vi "haotian_sheet_resistance.vi"() -> ()   [LabVIEW 2024]
uses:
  <vilib>/Utility/file.llb/Write Delimited Spreadsheet (DBL).vi
panel:
  out "Device 1 resistance":dbl=36696923.98728005
  out "Ch 1 phase":dbl=6.260435993401659 caption="Device1 phase" format="%.3p"
  out "Device1 Current(uA)":dbl=2.609667211877282
  in  "R1(Kohm)":dbl=2000.0 format="%#_13g"
  in  "path2 (folder + filename)":string="H:\\My Drive\\Lab\\PPMS\\Measurement\\GaN_1000C_3min_1314_1112"
  in  "Save data or not":bool=TRUE
  in  "path1 (folder + filename)":string="H:\\My Drive\\Lab\\PPMS\\Measurement\\GaN_1000C_2min_34_56"
  in  "V Loop#":i32=1
  out "Sine voltage T":dbl=1.0 format="%#_13g"
  out "Backward":bool
  out "Forward":bool=TRUE
  in  "V Step(mV)":i32=50
  out "V Loop Run T":i32=1
  in  "High Value (V)":dbl=5.0
  in  "Low Value (V)":dbl=1.0
  in  "System Stablization (s)":dbl=0.5 format="%#_13g"
  in  "LOCKIN1 address":refnum<visa-resource-name>="COM3"
  in  "A frequency":dbl=26.7 format="%#_13g"
  in  "A Input Connection (0: Single-Ended)":u16(ring)=1 items=["Single-Ended Voltage", "Differential Voltage", "1 MOhm Current Gain", "100 MOhm Current Gain"]
  in  "A harmonic 1":u8=2
  in  "A harmonic 2":u8=3
  in  "auto phase A":bool=TRUE
  in  "A Reference Source":u8(ring)=1 items=["External", "Internal", "Internal Sweep"]
  in  "A Sample time (s)":dbl=0.001 min=0.001 max=100.0 step=0.001
  in  "A Time Constant":u8(ring)=9 items=["10 us", "30 us", "100 us", "300 us", "1 ms", "3 ms", "10 ms", "30 ms", "100 ms", "300 ms", "1 s", "3 s", "10 s", "30 s", "100 s", "300 s", "1 ks", "3 ks"]
  in  "Enable Sync Filter A (open when f<200Hz)":bool
  in  "A Sensitivity":u16(ring)=26 items=["1 nV/fA", "2 nV/fA", "5 nV/fA", "10 nV/fA", "20 nV/fA", "50 nV/fA", "100 nV/fA", "200 nV/fA", "500 nV/fA", "1 uV/pA", "2 uV/pA", "5 uV/pA", "10 uV/pA", "20 uV/pA", "50 uV/pA", "100 uV/pA", "200 uV/pA", "500 uV/pA", "1 mV/nA", "2 mV/nA", "5 mV/nA", "10 mV/nA", "20 mV/nA", "50 mV/nA", "100 mV/nA", "200 mV/nA", "500 mV/nA", "1 V/uA"]
  in  "A Low Pass Filter Slope":u8(ring)=2 items=["6 dB/oct", "12 dB/oct", "18 db/oct", "24 dB/oct"]
  # "Statue"
  # "Ch1 Measurement"
  # "Lock-in Setting"
  # "Channel 1A"
  # "Sweep Setting"
  # "Channel 2A"
  # "Current Measurement"
  # "Channel 2B"
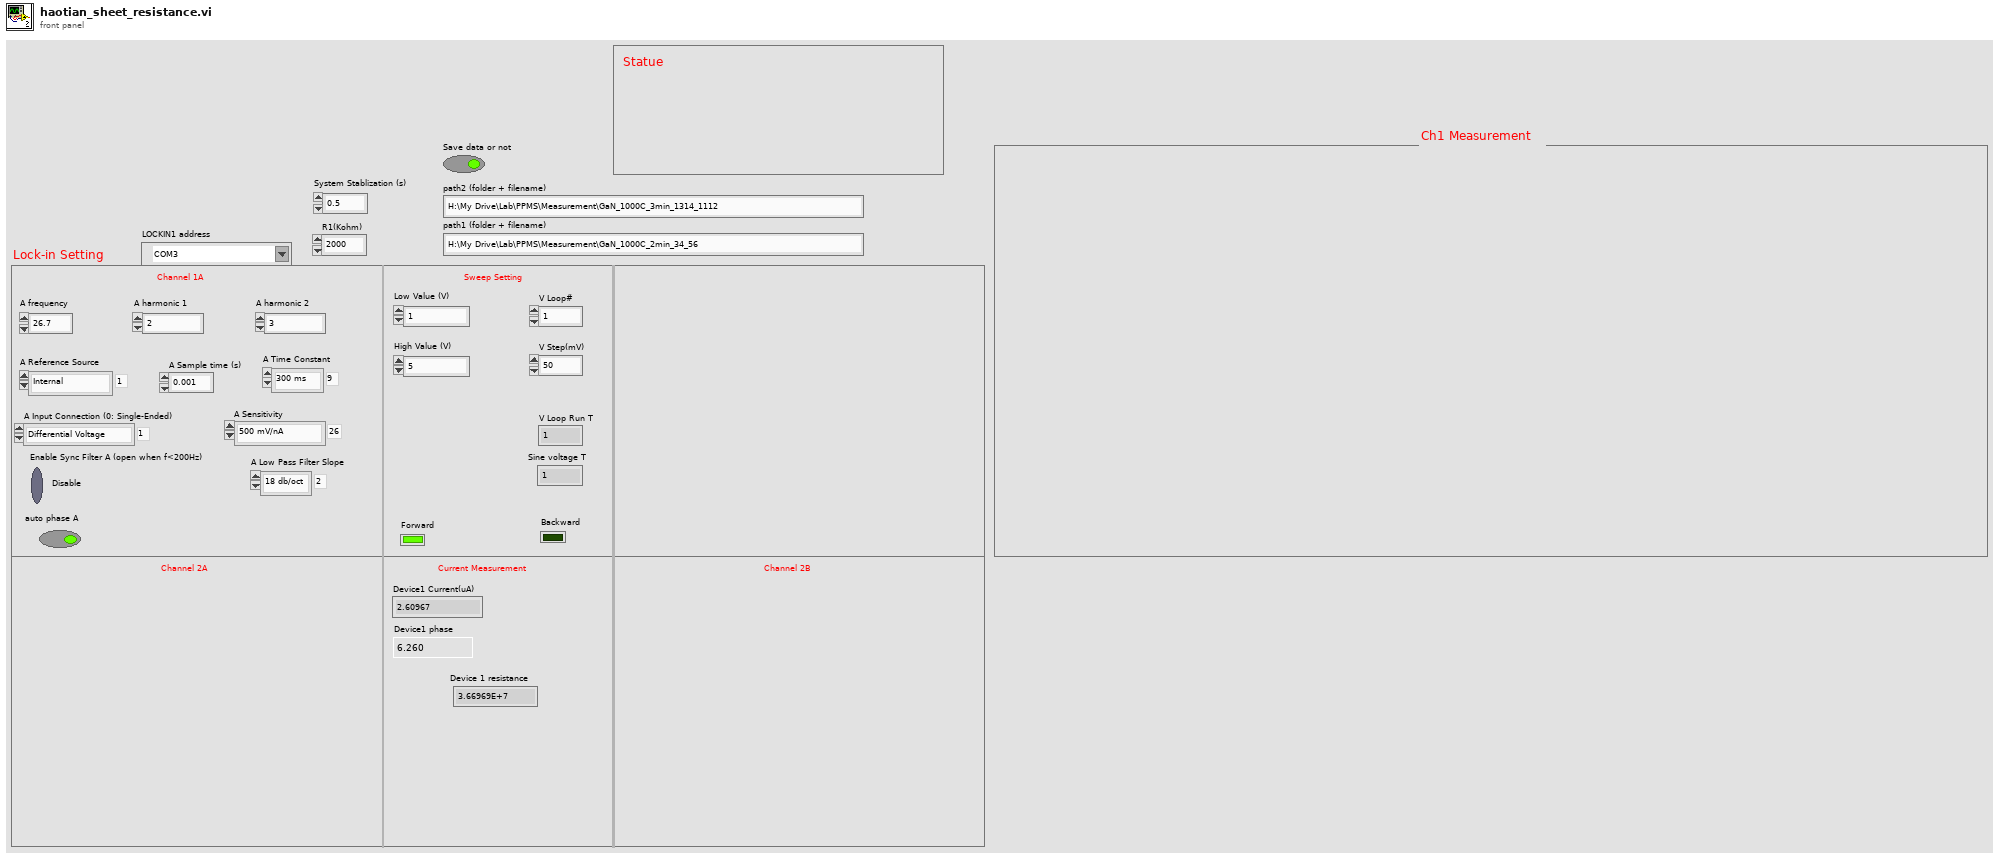
[diagram p1: front panel]
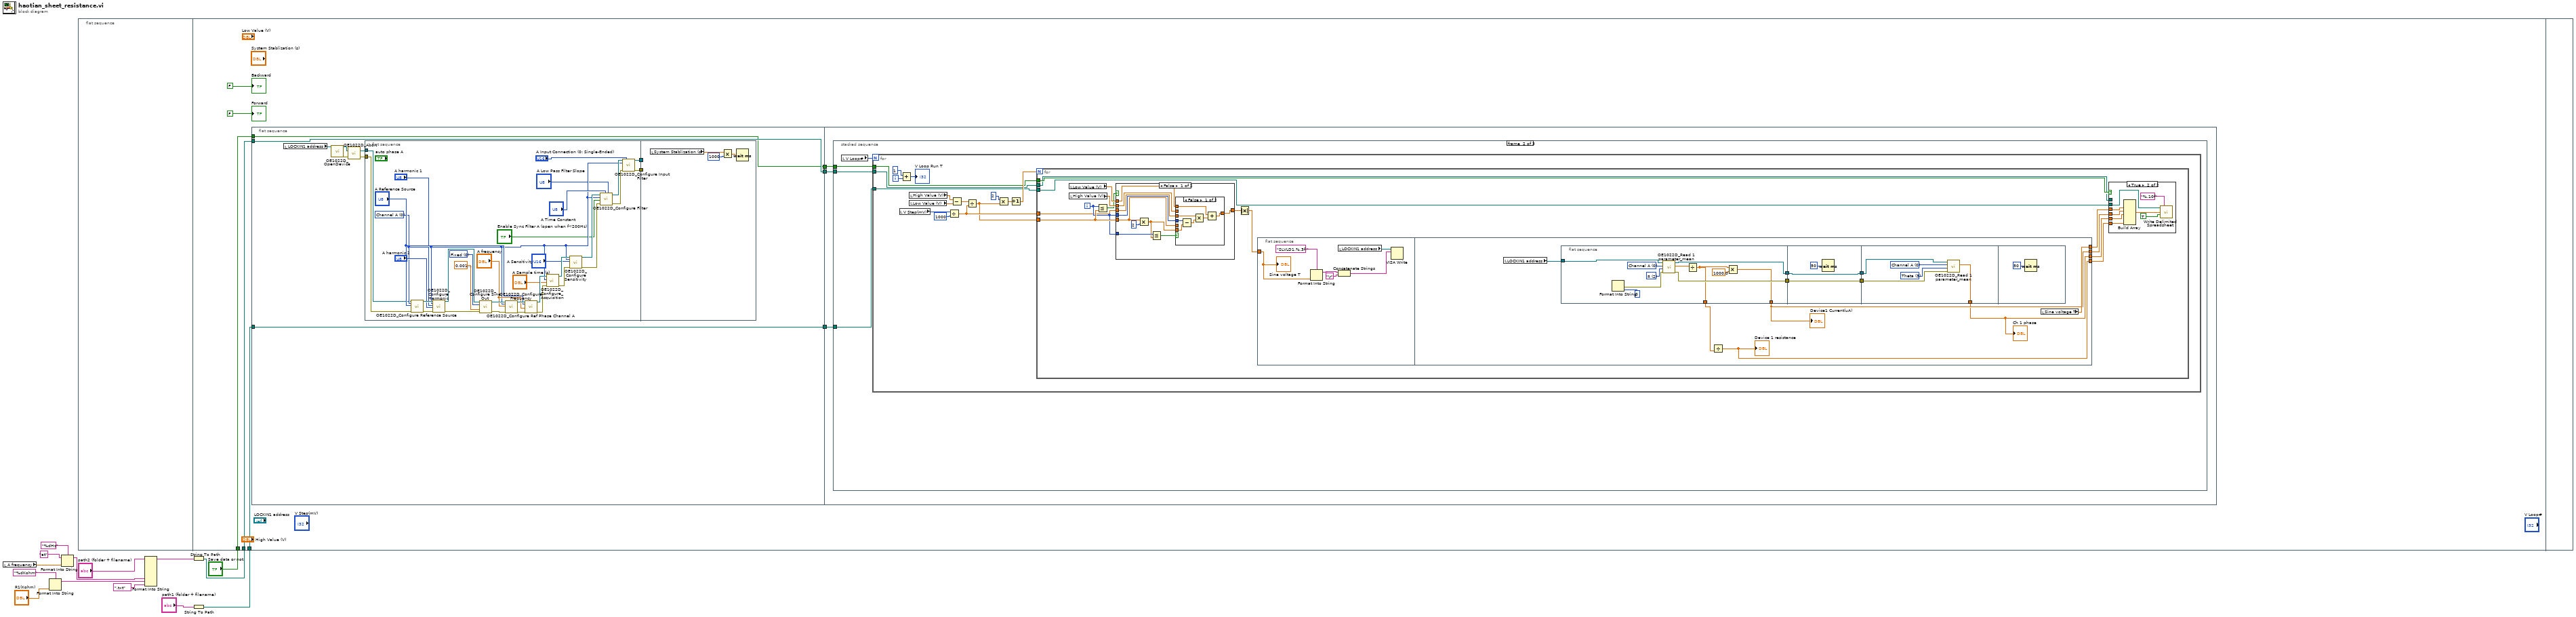
[diagram p0: block diagram]
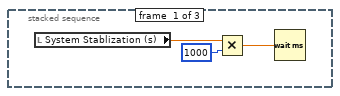
[diagram p2: hidden frame]
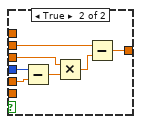
[diagram p3: hidden frame]
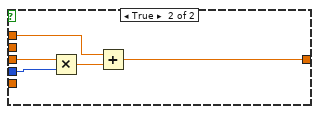
[diagram p4: hidden frame]
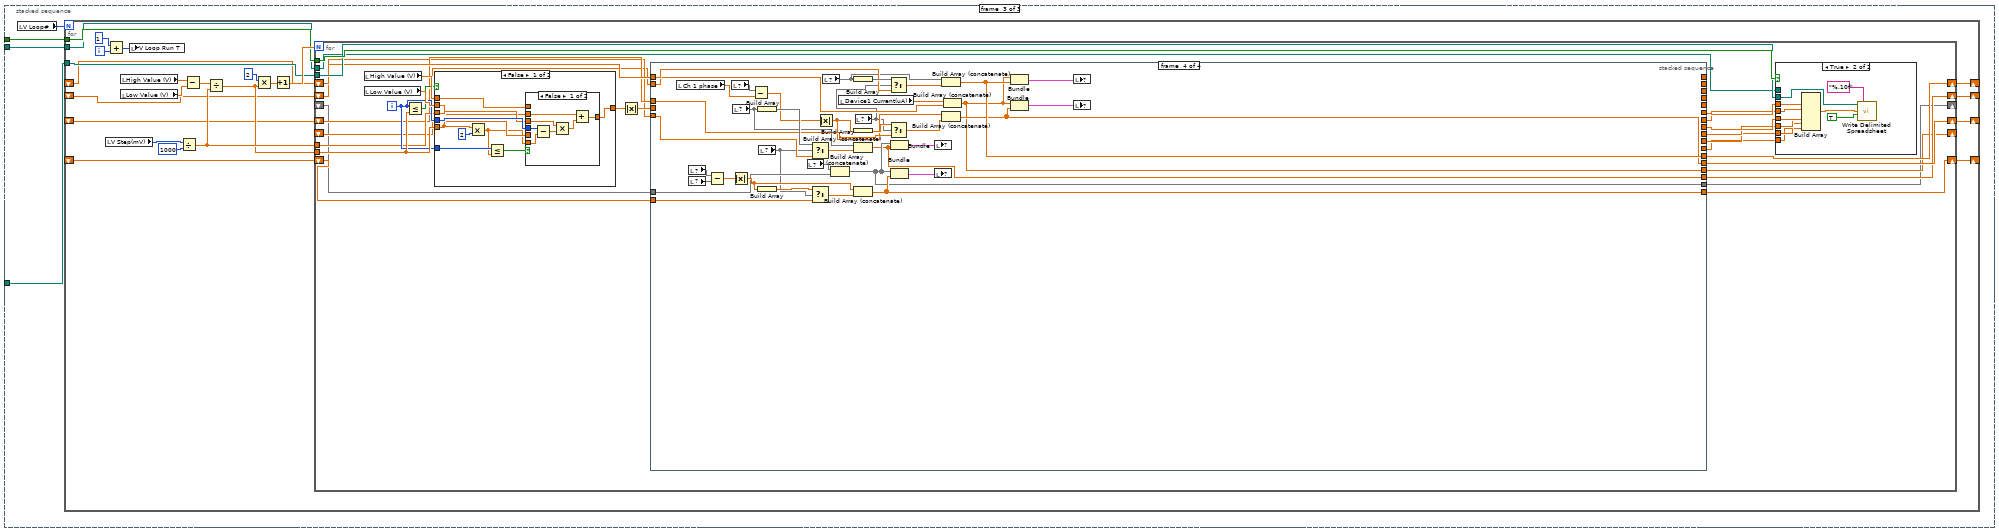
[diagram p6: hidden frame]
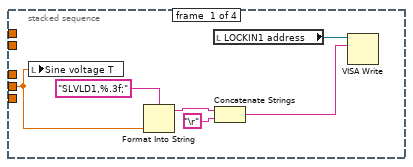
[diagram p7: hidden frame]
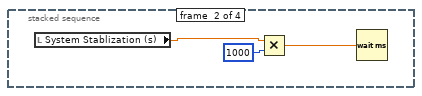
[diagram p8: hidden frame]
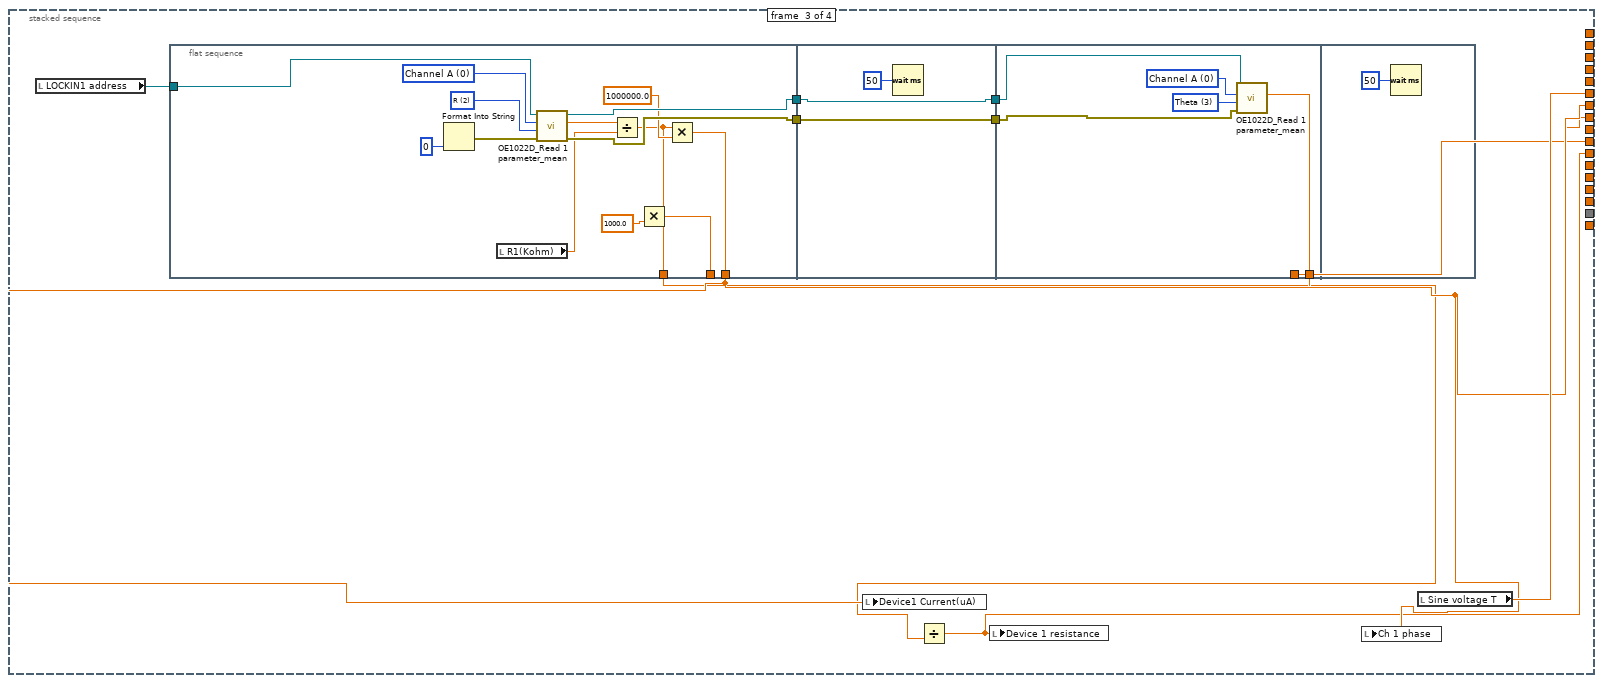
[diagram p9: hidden frame]
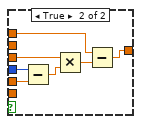
[diagram p10: hidden frame]
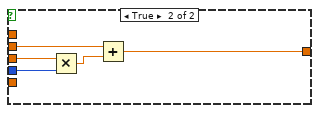
[diagram p11: hidden frame]
diagram:
  n1 = local read "A frequency"() -> (w13:dbl)
  n2 = Format Into String(format string="%dKohm", "R1(Kohm)") -> (resulting string=w1:string)  [unwired: 2 in, 1 out]
  n3 = Format Into String(format string="%dHz", initial string="at", w13) -> (resulting string=w9:string)  [unwired: 1 in, 1 out]
  n4 = flat-sequence {
    tunnel: w7 -> [w20]
    tunnel: w6 -> [w19]
    tunnel: "Save data or not" -> [w18]
    frame #0 {
    }
    frame #1 {
      n5 = flat-sequence {
        tunnel: w20 -> [w25]
        tunnel: [w25] -> w17
        tunnel: w19 -> [w24]
        tunnel: [w24] -> w16
        tunnel: w18 -> [w23]
        tunnel: [w23] -> w15
        tunnel: w17 -> [w70]
        tunnel: w16 -> [w69]
        tunnel: w15 -> [w71]
        frame #0 {
          n6 = local read "LOCKIN1 address"() -> (w27:refnum<visa-resource-name>)
          n7 = call "OE1022D_OpenDevice.vi"("VISA resource name"=w27) -> ("VISA资源名称输出"=w28:refnum<visa-resource-name>, "错误输出"=w29:errorcluster)  [unwired: 17 in]
          n8 = call "OE1022D_Abort.vi"("error in (no error)"=w29, "VISA resource name"=w28) -> ("error out"=w31:errorcluster, "VISA resource name out"=w32:refnum<visa-resource-name>)
          n9 = flat-sequence {
            tunnel: w32 -> [w33]
            tunnel: [w57] -> w30
            tunnel: w31 -> [w34]
            tunnel: [w35] -> w26
            tunnel: w30 -> [_]
            tunnel: w26 -> [_]
            frame #0 {
              w48 = u8 0 items=["Fixed", "Linear", "Log"] ("SineOut Mode")
              w39 = u8 0 items=["Channel A", "Channel B"] ("OE1022D A/B")
              n10 = call "OE1022D_Configure Reference Source.vi"("VISA resource name"=w33, "OE1022D A/B"=w39, "Reference Source"="A Reference Source", "error in (no error)"=w34) -> ("VISA resource name out"=w61:refnum<visa-resource-name>, "error out"=w59:errorcluster)  [unwired: 14 in]
              n11 = call "OE1022D_Configure Harmonic.vi"("VISA resource name"=w61, "OE1022D A/B"=w39, "Harmonic 1"="A harmonic 1", "Harmonic 2"="A harmonic 2", "error in (no error)"=w59) -> ("VISA resource name out"=w60:refnum<visa-resource-name>, "error out"=w58:errorcluster)  [unwired: 13 in]
              n12 = call "OE1022D_Configure Sine Out.vi"("VISA resource name"=w60, "SineOut Mode"=w48, "Sine Output Amplitude (V)"=sgl 0.001 ("A Sine Output Amplitude (V)"), "error in (no error)"=w58) -> ("VISA resource name out"=w64:refnum<visa-resource-name>, "error out"=w63:errorcluster)  [unwired: 10 in]
              n13 = call "OE1022D_Configure Frequency.vi"("VISA resource name"=w64, "OE1022D A/B"=w39, "Internal Frequency(Hz)"="A frequency", "error in (no error)"=w63) -> ("VISA resource name out"=w56:refnum<visa-resource-name>, "error out"=w53:errorcluster)  [unwired: 14 in]
              n14 = call "OE1022D_Configure Ref Phase Channel A.vi"("VISA resource name"=w56, "Reference Source"="A Reference Source", "Internal Frequency(Hz)"="A frequency", "error in (no error)"=w53) -> ("VISA resource name out"=w55:refnum<visa-resource-name>, "error out"=w54:errorcluster)  [unwired: 14 in]
              n15 = call "OE1022D_Configure_Acquisition.vi"("VISA resource name"=w55, "OE1022D A/B"=w39, "Sample time (s)"="A Sample time (s)", "error in (no error)"=w54) -> ("VISA resource name out"=w42:refnum<visa-resource-name>, "error out"=w41:errorcluster)  [unwired: 4 in]
              n16 = call "OE1022D_Configure Sensitivity.vi"("VISA resource name"=w42, "OE1022D A/B"=w39, "Sensitivity"="A Sensitivity", "error in (no error)"=w41) -> ("VISA resource name out"=w46:refnum<visa-resource-name>, "error out"=w45:errorcluster)  [unwired: 14 in]
              n17 = call "OE1022D_Configure Filter.vi"("Low Pass Filter Slope (1: 12dB/oct)"="A Low Pass Filter Slope", "Time Constant (8: 100ms)"="A Time Constant", "error in (no error)"=w45, "Enable Sync Filter (F: Disable)"="Enable Sync Filter A (open when f<200Hz)", "OE1022D A/B"=w39, "VISA resource name"=w46) -> ("error out"=w43:errorcluster, "VISA resource name out"=w44:refnum<visa-resource-name>)  [unwired: 4 in]
              n18 = call "OE1022D_Configure Input Filter.vi"("VISA resource name"=w44, "Input Source"="A Input Connection (0: Single-Ended)", "OE1022D A/B"=w39, "error in (no error)"=w43) -> ("VISA resource name out"=w35:refnum<visa-resource-name>, "error out"=w57:errorcluster)  [unwired: 10 in]
            }
            frame #1 {
              n19 = local read "System Stablization (s)"() -> (w66:dbl)
              n20 = Multiply(x=w66, y=1000) -> (x*y=w68:dbl)
              n21 = Wait (ms)(milliseconds to wait=w68) -> ()  [unwired: 1 out]
            }
          }
        }
        frame #1 {
          n22 = stacked-sequence {
            tunnel: w71 -> [_ w77 w185]
            tunnel: w70 -> [_ w76 w184]
            tunnel: w69 -> [_ w75 w183]
            frame #0 {
              n23 = local read "System Stablization (s)"() -> (w72:dbl)
              n24 = Multiply(x=w72, y=1000) -> (x*y=w74:dbl)
              n25 = Wait (ms)(milliseconds to wait=w74) -> ()  [unwired: 1 out]
            }
            frame #1 {
              n26 = local read "V Loop#"() -> (w78:i32)
              n27 = for {
                N: w78 -> [_]
                tunnel: w77 -> [w81]
                tunnel: w76 -> [w80]
                tunnel: w75 -> [w79]
                i -> [w94]
                n28 = local read "V Step(mV)"() -> (w82:i32)
                n29 = Add(x=1, y=w94) -> (x+y=→"V Loop Run T":i32)
                n30 = local read "High Value (V)"() -> (w84:dbl)
                n31 = local read "Low Value (V)"() -> (w83:dbl)
                n32 = Divide(x=w82, y=1000) -> (x/y=w86:dbl)
                n33 = Subtract(x=w84, y=w83) -> (x-y=w89:dbl)
                n34 = Divide(x=w89, y=w86) -> (x/y=w85:dbl)
                n35 = Multiply(x=2, y=w85) -> (x*y=w88:dbl)
                n36 = Increment(x=w88) -> (x+1=w87:dbl)
                n37 = for {
                  N: w87 -> [_]
                  tunnel: w86 -> [w104]
                  tunnel: w85 -> [w106]
                  tunnel: w81 -> [w101]
                  tunnel: w80 -> [w100]
                  tunnel: w79 -> [w99]
                  i -> [w105]
                  n38 = local read "Low Value (V)"() -> (w109:dbl)
                  n39 = local read "High Value (V)"() -> (w108:dbl)
                  n40 = Less Or Equal?(x=w105, y=w106) -> (x <= y?=w107:bool)
                  n41 = case shown="False" w107 {
                    tunnel: w109 -> [w146 w174]
                    tunnel: w105 -> [w155 w173]
                    tunnel: w104 -> [w154 w172]
                    tunnel: [w152 w170] -> w103
                    tunnel: w108 -> [w153 _]
                    tunnel: w106 -> [w148 _]
                    tunnel: w105 -> [w151 _]
                    frame False {
                      n42 = Multiply(x=w148, y=2) -> (x*y=w147:dbl)
                      n43 = Less Or Equal?(x=w151, y=w147) -> (x <= y?=w149:bool)
                      n44 = case shown="False" w149 {
                        tunnel: w155 -> [w162 w169]
                        tunnel: w154 -> [w160 w167]
                        tunnel: w153 -> [_ w165]
                        tunnel: [w158 w164] -> w152
                        tunnel: w148 -> [_ w163]
                        tunnel: w147 -> [w157 _]
                        tunnel: w146 -> [w156 _]
                        frame False {
                          n45 = Subtract(x=w162, y=w157) -> (x-y=w161:dbl)
                          n46 = Multiply(x=w160, y=w161) -> (x*y=w159:dbl)
                          n47 = Add(x=w156, y=w159) -> (x+y=w158:dbl)
                        }
                        frame True {
                          n48 = Subtract(x=w169, y=w163) -> (x-y=w168:dbl)
                          n49 = Multiply(x=w167, y=w168) -> (x*y=w166:dbl)
                          n50 = Subtract(x=w165, y=w166) -> (x-y=w164:dbl)
                        }
                      }
                    }
                    frame True {
                      n51 = Multiply(x=w172, y=w173) -> (x*y=w171:dbl)
                      n52 = Add(x=w174, y=w171) -> (x+y=w170:dbl)
                    }
                  }
                  n53 = Absolute Value(x=w103) -> (abs(x)=w102:dbl)
                  n54 = flat-sequence {
                    tunnel: w102 -> [w112]
                    tunnel: [w125] -> w98
                    tunnel: [w119] -> w97
                    tunnel: [w118] -> w96
                    tunnel: [w116] -> w95
                    frame #0 {
                      n55 = Format Into String(format string="SLVLD1,%.3f;", w112) -> (resulting string=w113:string)  [unwired: 2 in, 1 out]
                      n56 = local read "LOCKIN1 address"() -> (w111:refnum<visa-resource-name>)
                      n57 = Concatenate Strings(w113, "\r") -> (w110:string)
                      n58 = VISA Write(VISA resource name=w111, write buffer=w110) -> ()  [unwired: 1 in, 3 out]
                      "Sine voltage T" <- w112
                    }
                    frame #1 {
                      n59 = local read "LOCKIN1 address"() -> (w120:refnum<visa-resource-name>)
                      n60 = flat-sequence {
                        tunnel: w120 -> [w133]
                        tunnel: [w132] -> w124
                        tunnel: [w131] -> w123
                        tunnel: [w127] -> w119
                        tunnel: [w126] -> w117
                        tunnel: [w138] -> w122
                        tunnel: w124 -> [w138]
                        tunnel: w123 -> [w137]
                        tunnel: [w137] -> w121
                        tunnel: w122 -> [w144]
                        tunnel: w121 -> [w143]
                        tunnel: [w140] -> w118
                        frame #0 {
                          w130 = u16 2 items=["X", "Y", "R", "Theta", "Frequency", "Noise", "Xh1", "Yh1", "Rh1", "Theta h1", "Xh2", "Yh2", "Rh2", "Theta h2"] ("Parameter")
                          w134 = u16 0 items=["Channel A", "Channel B", "ADC"] ("Channel (0: A)")
                          n61 = Format Into String(0) -> (error out=w135:errorcluster)  [unwired: 3 in, 1 out]
                          n62 = call "OE1022D_Read 1 parameter_mean.vi"("错误输入（无错误）"=w135, "Parameter"=w130, "Channel (0: A)"=w134, "VISA resource name"=w133) -> ("error out"=w131:errorcluster, "Measurement"=w129:dbl, "VISA resource name out"=w132:refnum<visa-resource-name>)  [unwired: 5 in]
                          n63 = Divide(x=w129) -> (x/y=w126:dbl)  [unwired: 1 in]
                          n64 = Multiply(x=w126, y=1000.0) -> (x*y=w127:dbl)
                        }
                        frame #1 {
                          n65 = Wait (ms)(milliseconds to wait=u32 50) -> ()  [unwired: 1 out]
                        }
                        frame #2 {
                          w141 = u16 3 items=["X", "Y", "R", "Theta", "Frequency", "Noise", "Xh1", "Yh1", "Rh1", "Theta h1", "Xh2", "Yh2", "Rh2", "Theta h2"] ("Parameter")
                          w142 = u16 0 items=["Channel A", "Channel B", "ADC"] ("Channel (0: A)")
                          n66 = call "OE1022D_Read 1 parameter_mean.vi"("错误输入（无错误）"=w143, "Parameter"=w141, "Channel (0: A)"=w142, "VISA resource name"=w144) -> ("Measurement"=w140:dbl)  [unwired: 5 in, 2 out]
                        }
                        frame #3 {
                          n67 = Wait (ms)(milliseconds to wait=u32 50) -> ()  [unwired: 1 out]
                        }
                      }
                      n68 = Divide(y=w117) -> (x/y=w116:dbl)  [unwired: 1 in]
                      "Device 1 resistance" <- w116
                      n69 = local read "Sine voltage T"() -> (w125:dbl)
                      "Device1 Current(uA)" <- w119
                      "Ch 1 phase" <- w118
                    }
                  }
                  n70 = case shown="True" w101 {
                    tunnel: w98 -> [_ w176]
                    tunnel: w100 -> [_ w179]
                    tunnel: w99 -> [_ _]
                    tunnel: w97 -> [_ w178]
                    tunnel: w96 -> [_ w177]
                    tunnel: w95 -> [_ w175]
                    frame False {
                    }
                    frame True {
                      n71 = Build Array(w176, w178, w177, w175) -> (w181:dbl[])  [unwired: 4 in]
                      n72 = call-poly <vilib>:"Write Delimited Spreadsheet.vi"("file path (dialog if empty)"=w179, "format (%.3f)"="%.10f", "1D data"=w181, "append to file? (new file:F)"=TRUE) -> ()  [unwired: 10 in, 2 out]
                    }
                  }
                }
              }
            }
            frame #2 {
              n73 = local read "V Loop#"() -> (w186:i32)
              n74 = for {
                N: w186 -> [_]
                tunnel: w185 -> [w198]
                tunnel: w184 -> [w197]
                tunnel: w183 -> [w196]
                shift-right: [w195] -> _
                shift-left: _ -> [w194]
                shift-right: [w193] -> _
                shift-left: _ -> [w192]
                shift-right: [w191] -> _
                shift-left: _ -> [w190]
                shift-right: [w189] -> _
                shift-left: _ -> [w188]
                i -> [w210]
                n75 = local read "V Step(mV)"() -> (w199:i32)
                n76 = Add(x=1, y=w210) -> (x+y=w187:i32)
                n77 = local read "High Value (V)"() -> (w201:dbl)
                n78 = local read "Low Value (V)"() -> (w200:dbl)
                n79 = local write "V Loop Run T"(w187) -> ()
                n80 = Divide(x=w199, y=1000) -> (x/y=w203:dbl)
                n81 = Subtract(x=w201, y=w200) -> (x-y=w206:dbl)
                n82 = Divide(x=w206, y=w203) -> (x/y=w202:dbl)
                n83 = Multiply(x=2, y=w202) -> (x*y=w205:dbl)
                n84 = Increment(x=w205) -> (x+1=w204:dbl)
                n85 = for {
                  N: w204 -> [_]
                  tunnel: w203 -> [w234]
                  tunnel: w202 -> [w236]
                  tunnel: w198 -> [w231]
                  tunnel: w197 -> [w230]
                  tunnel: w196 -> [w229]
                  shift-right: [w227] -> w195
                  shift-left: w194 -> [w226]
                  shift-right: [w225] -> w193
                  shift-left: w192 -> [w224]
                  shift-right: [w223] -> w191
                  shift-left: w190 -> [w222]
                  shift-right: [w221] -> w189
                  shift-left: w188 -> [w220]
                  shift-right: [w215] -> _
                  shift-left: _ -> [w214]
                  shift-right: [w213] -> _
                  shift-left: _ -> [w212]
                  i -> [w235]
                  n86 = local read "High Value (V)"() -> (w238:dbl)
                  n87 = local read "Low Value (V)"() -> (w239:dbl)
                  n88 = Less Or Equal?(x=w235, y=w236) -> (x <= y?=w237:bool)
                  n89 = case shown="False" w237 {
                    tunnel: w239 -> [w327 w355]
                    tunnel: w235 -> [w336 w354]
                    tunnel: w234 -> [w335 w353]
                    tunnel: [w333 w351] -> w233
                    tunnel: w238 -> [w334 _]
                    tunnel: w236 -> [w329 _]
                    tunnel: w235 -> [w332 _]
                    frame False {
                      n90 = Multiply(x=w329, y=2) -> (x*y=w328:dbl)
                      n91 = Less Or Equal?(x=w332, y=w328) -> (x <= y?=w330:bool)
                      n92 = case shown="False" w330 {
                        tunnel: w336 -> [w343 w350]
                        tunnel: w335 -> [w341 w348]
                        tunnel: w334 -> [_ w346]
                        tunnel: [w339 w345] -> w333
                        tunnel: w329 -> [_ w344]
                        tunnel: w328 -> [w338 _]
                        tunnel: w327 -> [w337 _]
                        frame False {
                          n93 = Subtract(x=w343, y=w338) -> (x-y=w342:dbl)
                          n94 = Multiply(x=w341, y=w342) -> (x*y=w340:dbl)
                          n95 = Add(x=w337, y=w340) -> (x+y=w339:dbl)
                        }
                        frame True {
                          n96 = Subtract(x=w350, y=w344) -> (x-y=w349:dbl)
                          n97 = Multiply(x=w348, y=w349) -> (x*y=w347:dbl)
                          n98 = Subtract(x=w346, y=w347) -> (x-y=w345:dbl)
                        }
                      }
                    }
                    frame True {
                      n99 = Multiply(x=w353, y=w354) -> (x*y=w352:dbl)
                      n100 = Add(x=w355, y=w352) -> (x+y=w351:dbl)
                    }
                  }
                  n101 = Absolute Value(x=w233) -> (abs(x)=w232:dbl)
                  n102 = stacked-sequence {
                    tunnel: w232 -> [w240 _ _ _]
                    tunnel: [_ _ w265 _] -> w228
                    tunnel: [_ _ _ w318] -> w227
                    tunnel: w226 -> [_ _ _ w317]
                    tunnel: [_ _ _ w316] -> w225
                    tunnel: w224 -> [_ _ _ w315]
                    tunnel: [_ _ _ w299] -> w223
                    tunnel: w222 -> [_ _ _ w314]
                    tunnel: [_ _ _ w313] -> w221
                    tunnel: w220 -> [_ _ _ w312]
                    tunnel: [_ _ w257 _] -> w216
                    tunnel: [_ _ w259 _] -> w219
                    tunnel: [_ _ w258 _] -> w218
                    tunnel: [_ _ _ _] -> w217
                    tunnel: _ -> [_ _ w256 _]
                    tunnel: _ -> [_ _ w255 _]
                    tunnel: _ -> [_ _ w254 _]
                    tunnel: _ -> [_ _ w253 _]
                    tunnel: [_ _ _ w303] -> w215
                    tunnel: w214 -> [_ _ _ w302]
                    tunnel: [_ _ _ w301] -> w213
                    tunnel: w212 -> [_ _ _ w300]
                    tunnel: _ -> [_ _ w251 _]
                    tunnel: [_ _ w250 _] -> w211
                    frame #0 {
                      n103 = local write "Sine voltage T"(w240) -> ()
                      n104 = Format Into String(format string="SLVLD1,%.3f;", w240) -> (resulting string=w243:string)  [unwired: 2 in, 1 out]
                      n105 = local read "LOCKIN1 address"() -> (w242:refnum<visa-resource-name>)
                      n106 = Concatenate Strings(w243, "\r") -> (w241:string)
                      n107 = VISA Write(VISA resource name=w242, write buffer=w241) -> ()  [unwired: 1 in, 3 out]
                    }
                    frame #1 {
                      n108 = local read "System Stablization (s)"() -> (w246:dbl)
                      n109 = Multiply(x=w246, y=1000) -> (x*y=w248:dbl)
                      n110 = Wait (ms)(milliseconds to wait=w248) -> ()  [unwired: 1 out]
                    }
                    frame #2 {
                      n111 = local read "LOCKIN1 address"() -> (w260:refnum<visa-resource-name>)
                      n112 = flat-sequence {
                        tunnel: w260 -> [w276]
                        tunnel: [w275] -> w264
                        tunnel: [w274] -> w263
                        tunnel: [w267] -> w259
                        tunnel: [w269] -> _
                        tunnel: [w266] -> w252
                        tunnel: [w281] -> w262
                        tunnel: w264 -> [w281]
                        tunnel: w263 -> [w280]
                        tunnel: [w280] -> w261
                        tunnel: w262 -> [w287]
                        tunnel: w261 -> [w286]
                        tunnel: [w283] -> w258
                        tunnel: [_] -> w257
                        frame #0 {
                          w273 = u16 2 items=["X", "Y", "R", "Theta", "Frequency", "Noise", "Xh1", "Yh1", "Rh1", "Theta h1", "Xh2", "Yh2", "Rh2", "Theta h2"] ("Parameter")
                          w277 = u16 0 items=["Channel A", "Channel B", "ADC"] ("Channel (0: A)")
                          n113 = Format Into String(0) -> (error out=w278:errorcluster)  [unwired: 3 in, 1 out]
                          n114 = local read "R1(Kohm)"() -> (w270:dbl)
                          n115 = call "OE1022D_Read 1 parameter_mean.vi"("错误输入（无错误）"=w278, "Parameter"=w273, "Channel (0: A)"=w277, "VISA resource name"=w276) -> ("error out"=w274:errorcluster, "Measurement"=w272:dbl, "VISA resource name out"=w275:refnum<visa-resource-name>)  [unwired: 5 in]
                          n116 = Divide(x=w272, y=w270) -> (x/y=w266:dbl)
                          n117 = Multiply(y=1000.0) -> (x*y=w269:dbl)  [unwired: 1 in]
                          n118 = Multiply(x=w266, y=1000000.0) -> (x*y=w267:dbl)
                        }
                        frame #1 {
                          n119 = Wait (ms)(milliseconds to wait=u32 50) -> ()  [unwired: 1 out]
                        }
                        frame #2 {
                          w284 = u16 3 items=["X", "Y", "R", "Theta", "Frequency", "Noise", "Xh1", "Yh1", "Rh1", "Theta h1", "Xh2", "Yh2", "Rh2", "Theta h2"] ("Parameter")
                          w285 = u16 0 items=["Channel A", "Channel B", "ADC"] ("Channel (0: A)")
                          n120 = call "OE1022D_Read 1 parameter_mean.vi"("错误输入（无错误）"=w286, "Parameter"=w284, "Channel (0: A)"=w285, "VISA resource name"=w287) -> ("Measurement"=w283:dbl)  [unwired: 5 in, 2 out]
                        }
                        frame #3 {
                          n121 = Wait (ms)(milliseconds to wait=u32 50) -> ()  [unwired: 1 out]
                        }
                      }
                      n122 = local write "Device1 Current(uA)"(w259) -> ()
                      n123 = Divide(y=w252) -> (x=w249:dbl, x/y=w250:dbl)
                      n124 = local write "Device 1 resistance"(w250) -> ()
                      n125 = local write "Ch 1 phase"(w258) -> ()
                      n126 = local read "Sine voltage T"() -> (w265:dbl)
                    }
                    frame #3 {
                      n127 = local read "Ch 1 phase"() -> (w309:dbl)
                      n128 = local read item#-1() -> (w306)
                      n129 = local read item#-1() -> (w305)
                      n130 = Subtract(x=w306, y=w305) -> (x-y=w307:dbl)
                      n131 = local read item#-1() -> (w308)
                      n132 = Absolute Value(x=w307) -> (abs(x)=w304:dbl)
                      n133 = local read item#-1() -> (w289)
                      n134 = Subtract(x=w308, y=w309) -> (x-y=w311:dbl)
                      n135 = Build Array(w289) -> (w325:void[])
                      n136 = Build Array(w304) -> (w321:dbl[])
                      n137 = local read item#-1() -> (w293)
                      n138 = local read item#-1() -> (w290)
                      n139 = Select(t=w325, s=w293, f=w314) -> (s? t:f=w319:dbl[])
                      n140 = Select(t=w321, s=w293, f=w312) -> (s? t:f=w320:dbl[])
                      n141 = Absolute Value(x=w311) -> (abs(x)=w310:dbl)
                      n142 = local read item#-1() -> (w292)
                      n143 = Build Array (concatenate)(w290, w300) -> (w301:void[])
                      n144 = local read "Device1 Current(uA)"() -> (w291:dbl)
                      n145 = Build Array(w292) -> (w326:void[])
                      n146 = Build Array(w310) -> (w323:dbl[])
                      n147 = Build Array (concatenate)(w289, w319) -> (w299:dbl[])
                      n148 = Build Array (concatenate)(w304, w320) -> (w313:dbl[])
                      n149 = local read item#-1() -> (w294)
                      n150 = Select(t=w326, s=w294, f=w317) -> (s? t:f=w324:dbl[])
                      n151 = Select(t=w323, s=w294, f=w315) -> (s? t:f=w322:dbl[])
                      n152 = Bundle(w301, w299) -> (w295:cluster{void[], dbl[]})  [unwired: 1 in]
                      n153 = Bundle(w301, w313) -> (w296:cluster{void[], dbl[]})  [unwired: 1 in]
                      n154 = local write item#-1(w295) -> ()
                      n155 = local write item#-1(w296) -> ()
                      n156 = Build Array (concatenate)(w292, w324) -> (w318:dbl[])
                      n157 = Build Array (concatenate)(w310, w322) -> (w316:dbl[])
                      n158 = Build Array (concatenate)(w291, w302) -> (w303:dbl[])
                      n159 = Bundle(w303, w318) -> (w298:cluster{dbl[], dbl[]})  [unwired: 1 in]
                      n160 = Bundle(w303, w316) -> (w297:cluster{dbl[], dbl[]})  [unwired: 1 in]
                      n161 = local write item#-1(w298) -> ()
                      n162 = local write item#-1(w297) -> ()
                    }
                  }
                  n163 = case shown="True" w231 {
                    tunnel: w228 -> [_ w357]
                    tunnel: w230 -> [_ w362]
                    tunnel: w229 -> [_ _]
                    tunnel: w219 -> [_ w361]
                    tunnel: w218 -> [_ w360]
                    tunnel: w217 -> [_ w359]
                    tunnel: w216 -> [_ w358]
                    tunnel: w211 -> [_ w356]
                    frame False {
                    }
                    frame True {
                      n164 = Build Array(w357, w361, w360, w359, w358, w356) -> (w364:dbl[])  [unwired: 2 in]
                      n165 = call-poly <vilib>:"Write Delimited Spreadsheet.vi"("file path (dialog if empty)"=w362, "format (%.3f)"="%.10f", "1D data"=w364, "append to file? (new file:F)"=TRUE) -> ()  [unwired: 10 in, 2 out]
                    }
                  }
                }
              }
            }
          }
        }
      }
      "Forward" <- FALSE ("Up")
      "Backward" <- FALSE ("Down")
    }
    frame #2 {
    }
  }
  n166 = Format Into String(initial string="path2 (folder + filename)", w9, w1, ".txt") -> (resulting string=w14:string)  [unwired: 6 in, 1 out]
  n167 = String To Path(string=w14) -> (path=w6:path)
  n168 = String To Path(string="path1 (folder + filename)") -> (path=w7:path)
